vi "Make DLL Param(Read Batch Profile Storage Rsp).vi"(1 "Read Batch Profile Storage Rsp":T2) -> (0 "pRsp":T1)   [LabVIEW 8.6, in "Keyence LJ-V7000.lvlib"]
uses:
  Keyence LJ-V7000.lvlib
  Public/Clusters/Time.ctl
  Public/Clusters/Read Batch Profile Storage Rsp.ctl
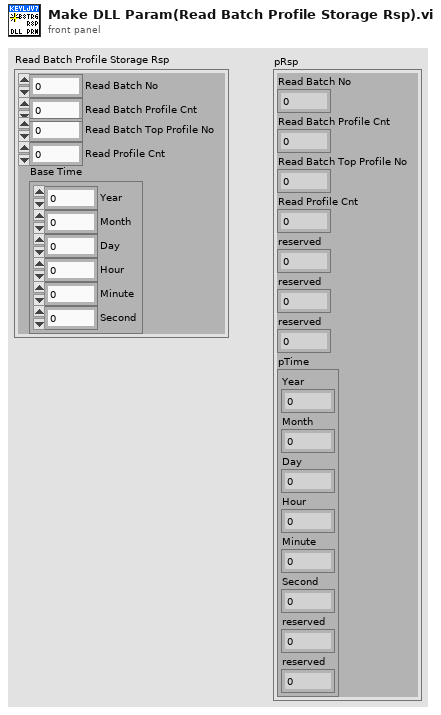
[diagram p1: front panel]
types:
  T1 = cluster{"Read Batch No":u32, "Read Batch Profile Cnt":u32, "Read Batch Top Profile No":u32, "Read Profile Cnt":u8, "reserved":u8, "reserved":u8, "reserved":u8, "pTime":cluster{"Year":u8, "Month":u8, "Day":u8, "Hour":u8, "Minute":u8, "Second":u8, "reserved":u8, "reserved":u8}}
  T2 = typedef "Keyence LJ-V7000.lvlib/Read Batch Profile Storage Rsp.ctl" = cluster{"Read Batch No":u32, "Read Batch Profile Cnt":u32, "Read Batch Top Profile No":u32, "Read Profile Cnt":u8, "Base Time":T3}
  T3 = typedef "Keyence LJ-V7000.lvlib/Time.ctl" = cluster{"Year":u8, "Month":u8, "Day":u8, "Hour":u8, "Minute":u8, "Second":u8}
  T4 = cluster{"Year":u8, "Month":u8, "Day":u8, "Hour":u8, "Minute":u8, "Second":u8, "reserved":u8, "reserved":u8}
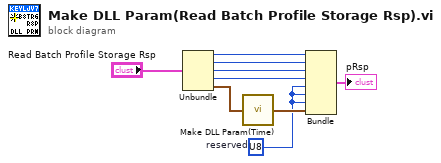
[diagram p0: block diagram]
diagram:
  w2 = u8 ?  # reserved
  n1 = Unbundle("Read Batch Profile Storage Rsp") -> ("Read Batch No"=w7:u32, "Read Batch Profile Cnt"=w6:u32, "Read Batch Top Profile No"=w5:u32, "Read Profile Cnt"=w4:u8, "Base Time"=w8:T3)
  n2 = call "Make DLL Param(Time).vi"("Time"=w8) -> ("pTime"=w3:T4)
  n3 = Bundle("Read Batch No"=w7, "Read Batch Profile Cnt"=w6, "Read Batch Top Profile No"=w5, "Read Profile Cnt"=w4, "reserved"=w2, "reserved"=w2, "reserved"=w2, "pTime"=w3) -> (→"pRsp":T1)  [unwired: 1 in]
